vi "Fc_to_CS_Enable.vi"(8 "error in (no error)":errorcluster, 9 "Class TCP":T1, 10 "CS_IF_Params":T2, 11 "CTRL enable":bool) -> (0 "error out":errorcluster)   [LabVIEW 2022 SP3]
doc: "This function enables the control system."
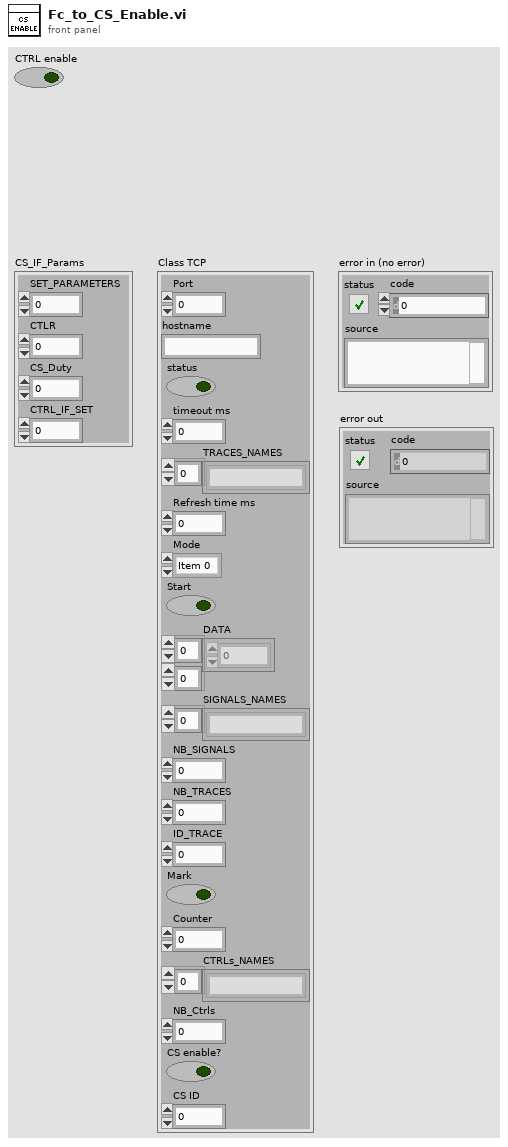
[diagram p1: front panel]
types:
  T1 = cluster{"Port":i32, "hostname":string, "status":bool, "timeout ms":i32, "TRACES_NAMES":string[], "Refresh time ms":i32, "Mode":enum32{"Item 0", "Item 1"}, "Start":bool, "DATA":sgl[][], "SIGNALS_NAMES":string[], "NB_SIGNALS":i32, "NB_TRACES":i32, "ID_TRACE":i32, "Mark":bool, "Counter":i32, "CTRLs_NAMES":string[], "NB_Ctrls":i32, "CS enable?":bool, "CS ID":i32}
  T2 = cluster{"SET_PARAMETERS":i32, "CTLR":i32, "CS_Duty":sgl, "CTRL_IF_SET":i32}
  T3 = cluster{"timeout ms":i32, "remote port":u16, "Address":string}
  T4 = cluster{"TRACE_SIZE":i32, "CS_ID":i32, "TRACE ID":i32, "CMD":i32, "DATA PARAM":string}
  T5 = enum16{"big-endian, network order", "native, host order", "little-endian"}
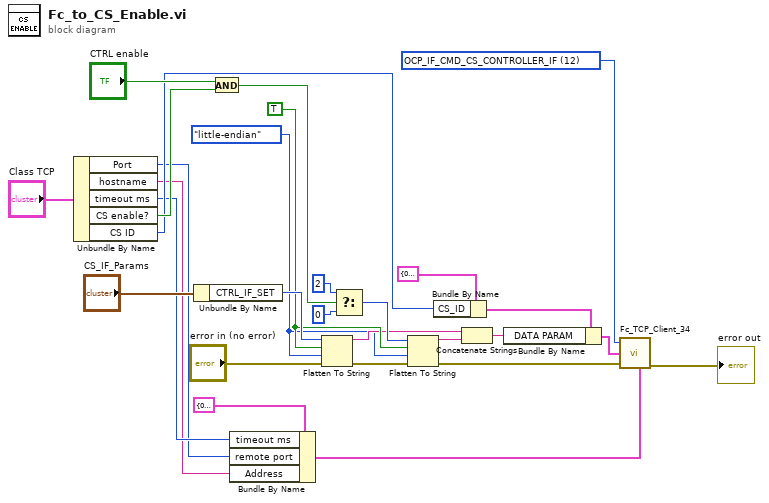
[diagram p0: block diagram]
diagram:
  w22 = TRUE
  w15 = 12 items=["OCP_IF_CMD_TRACE_READ", "OCP_IF_CMD_TRACE_RESET", "OCP_IF_CMD_TRACE_GET_SIZE", "OCP_IF_CMD_TRACE_SET_SIZE", "OCP_IF_CMD_TRACE_GET_NUMBER_SIGNALS", "OCP_IF_CMD_TRACE_GET_SIGNALS_NAMES", "OCP_IF_CMD_TRACE_GET_NUMBER_TRACES", "OCP_IF_CMD_TRACE_GET_TRACES_NAMES", "OCP_IF_CMD_TRACE_GET_ADDRESS", "OCP_IF_CMD_CS_STATUS", "OCP_IF_CMD_CS_ENABLE", "OCP_IF_CMD_CS_DISABLE", "OCP_IF_CMD_CS_CONTROLLER_IF", "OCP_IF_CMD_CS_HARDWARE_IF", "OCP_IF_CMD_CS_GET_NUMBER_CONTROLLERS", "OCP_IF_CMD_CS_GET_CONTROLLERS_NAMES", "OCP_IF_CMD_PLATFORM_ID", "OCP_IF_CMD_PLATFORM_IF", "OCP_IF_CMD_OPIL_UPDATE_MEASUREMENTS", "OCP_IF_CMD_OPIL_UPDATE_SIM_DATA", "OCP_IF_CMD_OPIL_RUN_CONTROL", "OCP_IF_CMD_OPIL_INITIALIZE_CONTROL", "OCP_IF_CMD_OPIL_GET_CONTROL", "OCP_IF_CMD_OPIL_GET_CONTROLLER_DATA", "OCP_IF_CMD_END"] ("CMD")
  w9 = T5."little-endian" ("byte order (0:big-endian, network order)")
  n1 = Unbundle By Name("Class TCP") -> ("Port"=w4:i32, "hostname"=w5:string, "timeout ms"=w6:i32, "CS enable?"=w11:bool, "CS ID"=w10:i32)
  n2 = Unbundle By Name("CS_IF_Params") -> ("CTRL_IF_SET"=w23:i32)
  n3 = And(x="CTRL enable", y=w11) -> (x .and. y?=w24:bool)
  n4 = Bundle By Name(cluster=T3 {"timeout ms"=0, "remote port"=0, "Address"=""} ("Comunication Cluster"), "timeout ms"=w6, "remote port"=w4, "Address"=w5) -> (w7:T3)
  n5 = Flatten To String(anything=w23, prepend array or string size? (T)=w22, byte order (0:big-endian, network order)=w9, error in (no error)="error in (no error)") -> (data string=w17:string, error out=w16:errorcluster)  [unwired: 1 out]
  n6 = Select(t=2 ("CTRL_IF_SET"), s=w24, f=0 ("CTRL_IF_SET")) -> (s? t:f=w26:i32)
  n7 = Flatten To String(anything=w26, prepend array or string size? (T)=w22, byte order (0:big-endian, network order)=w9, error in (no error)=w16) -> (data string=w18:string, error out=w19:errorcluster)  [unwired: 1 out]
  n8 = Bundle By Name(cluster=T4 {"TRACE_SIZE"=0, "CS_ID"=0, "TRACE ID"=0, "CMD"=0, "DATA PARAM"=""} ("Input Cluster"), "CS_ID"=w10) -> (w13:T4)
  n9 = Concatenate Strings(w17, w18) -> (w20:string)
  n10 = Bundle By Name(cluster=w13, "DATA PARAM"=w20) -> (w21:T4)
  n11 = call "Fc_TCP_Client_34.vi"("CMD"=w15, "Input Cluster"=w21, "error in (no error)"=w19, "Comunication Cluster"=w7) -> ("error out"=→"error out":errorcluster)  [unwired: 4 in, 2 out]
